vi "F Dwf Analog Out Symmetry Set.vi"(8 "error in (no error)":errorcluster, 9 "percentageSymmetry":dbl, 10 "idxChannel":i32, 11 "hdwf":i32) -> (0 "error out":errorcluster, 3 "function return":i32)   [LabVIEW 2019, in "Olasdwf.lvlib"]
doc: "DWFAPI int FDwfAnalogOutSymmetrySet(HDWF hdwf, int idxChannel, double percentageSymmetry);"
uses:
  Olasdwf.lvlib
  Windows/System32/dwf.dll
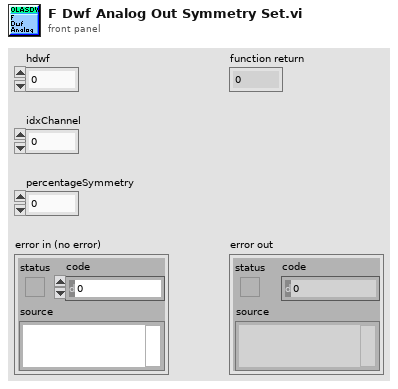
[diagram p1: front panel]
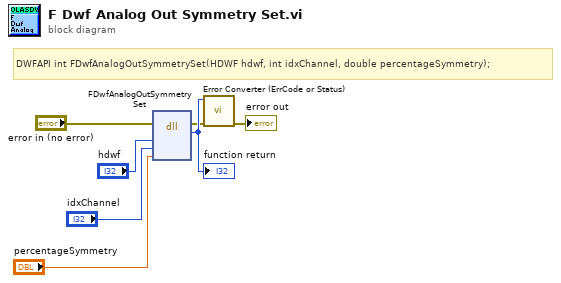
[diagram p0: block diagram]
diagram:
  # "DWFAPI int FDwfAnalogOutSymmetrySet(HDWF hdwf, int idxChannel, double percentageSymmetry);"
  n1 = dll-call lib="C:/Windows/System32/dwf.*" fn="FDwfAnalogOutSymmetrySet"(error in="error in (no error)", "hdwf"="hdwf", "idxChannel"="idxChannel", "percentageSymmetry"="percentageSymmetry") -> (error out=w2:errorcluster, w7:i32)  [unwired: 5 in, 1 out]
  "function return" <- w7
  n2 = call "Error Converter (ErrCode or Status).vi"("error in (no error)"=w2, "error code"=w7) -> ("error out"=→"error out":errorcluster)  [unwired: 9 in]
